vi "Is Complete.vi"(8 "error in (no error)":errorcluster, 11 "IV in":refnum<class "IV.lvclass">) -> (0 "error out":errorcluster, 2 "Is complete?":bool, 3 "IV out":refnum<class "IV.lvclass">)   [LabVIEW 2021, in "IV.lvclass"]
uses:
  IV.lvclass
  IV.lvclass/IV.ctl
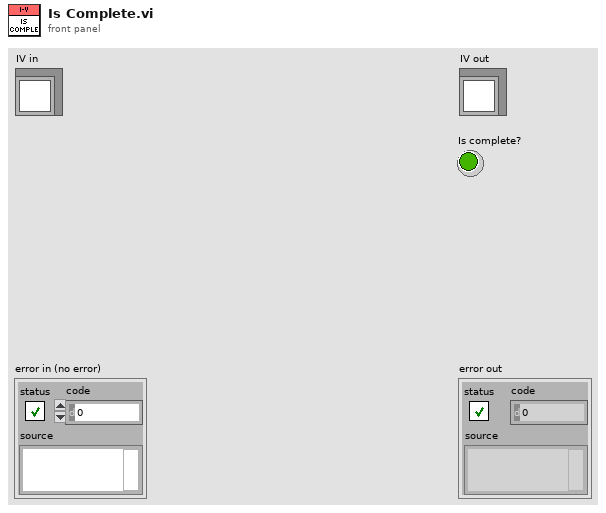
[diagram p1: front panel]
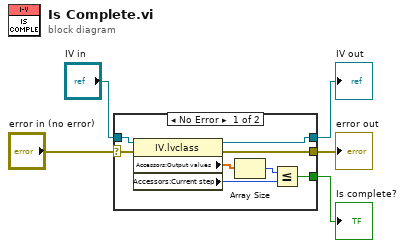
[diagram p0: block diagram]
diagram:
  n1 = case shown="No Error" "error in (no error)" {
    selector: "error in (no error)" -> [w13 w15]
    tunnel: [w12 w15] -> w4
    tunnel: [w10 w14] -> w2
    tunnel: "IV in" -> [w11 w14]
    tunnel: [w6 _] -> w1
    frame No Error {
      n2 = property class="IV.lvclass"(reference=w11, error in=w13) -> (reference out=w10:refnum<class "IV.lvclass">, error out=w12:errorcluster, "Accessors:Output values"=w9:dbl[], "Accessors:Current step"=w7:i32)
      n3 = Array Size(array=w9) -> (size(s)=w8:i32)
      n4 = Less Or Equal?(x=w8, y=w7) -> (x <= y?=w6:bool)
    }
    frame Error {
    }
  }
  "error out" <- w4
  "IV out" <- w2
  "Is complete?" <- w1
